vi "Keithley 2400 Init.vi"(8 "error in (no error)":errorcluster, 10 "Reset (True)":bool=TRUE, 11 "VISA Refnum in":refnum<visa-resource-name>) -> (0 "error out":errorcluster, 3 "VISA Refnum out":refnum<visa-resource-name>)   [LabVIEW 2019]
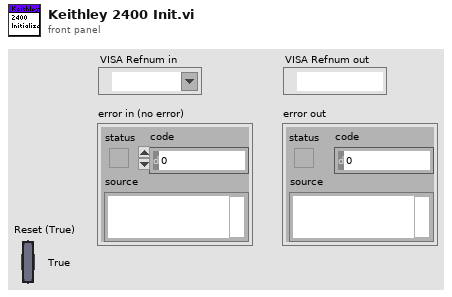
[diagram p1: front panel]
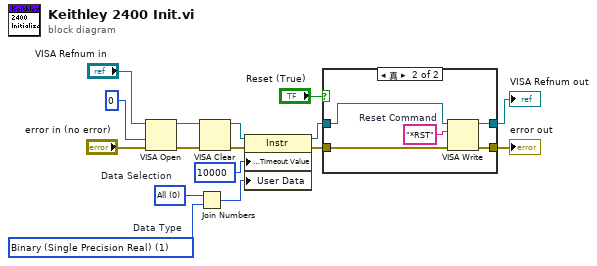
[diagram p0: block diagram]
diagram:
  w8 = u16 1 items=["ASCII", "Binary (Single Precision Real)"]  # Data Type
  w9 = u16 0 items=["All", "Volt and Amp", "Volt", "Amp"]  # Data Selection
  n1 = VISA Open(access mode=u32 0, error in (no error)="error in (no error)", VISA resource name="VISA Refnum in") -> (VISA resource name=w13:refnum<visa-resource-name>, error out=w12:errorcluster)  [unwired: 2 in]
  n2 = Join Numbers(hi=w9, lo=w8) -> ((hi.lo)=w7:u32)
  n3 = VISA Clear(VISA resource name=w13, error in (no error)=w12) -> (VISA resource name out=w11:refnum<visa-resource-name>, error out=w10:errorcluster)
  n4 = property class="Instr"(reference=w11, error in=w10, "General Settings:Timeout Value"=u32 10000, "User Data"=w7) -> (reference out=w4:refnum<visa-resource-name>, error out=w2:errorcluster)
  n5 = case shown="真" "Reset (True)" {
    tunnel: w4 -> [w18 w22]
    tunnel: [w18 w21] -> w3
    tunnel: w2 -> [w17 w20]
    tunnel: [w17 w19] -> w1
    frame False {
    }
    frame True {
      w23 = "*RST"  # Reset Command
      n6 = VISA Write(VISA resource name=w22, write buffer=w23, error in (no error)=w20) -> (VISA resource name out=w21:refnum<visa-resource-name>, error out=w19:errorcluster)  [unwired: 1 out]
    }
  }
  "error out" <- w1
  "VISA Refnum out" <- w3
